vi "K线诊断.vi"(9 "K线诊断":string[][](table)=[["ATI", "MW60K 190630 V3.3"], ["ATSP5", "ISO14230 FastInit"], ["ATSH8131F1", "OK"], ["8100", "7F 81 13"]], 10 "波特率":u32=38400, 11 "VISA resource name":refnum<visa-resource-name> caption="COM") -> (2 "字符串":string, 3 "逻辑与":bool)   [LabVIEW 2020]
uses:
  <vilib>/Instr/_visa.llb/VISA Configure Serial Port (Instr).vi
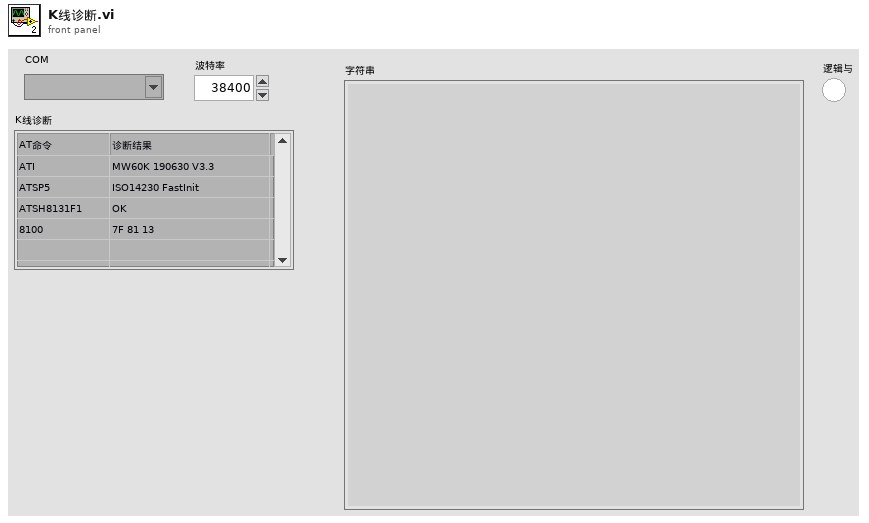
[diagram p1: front panel]
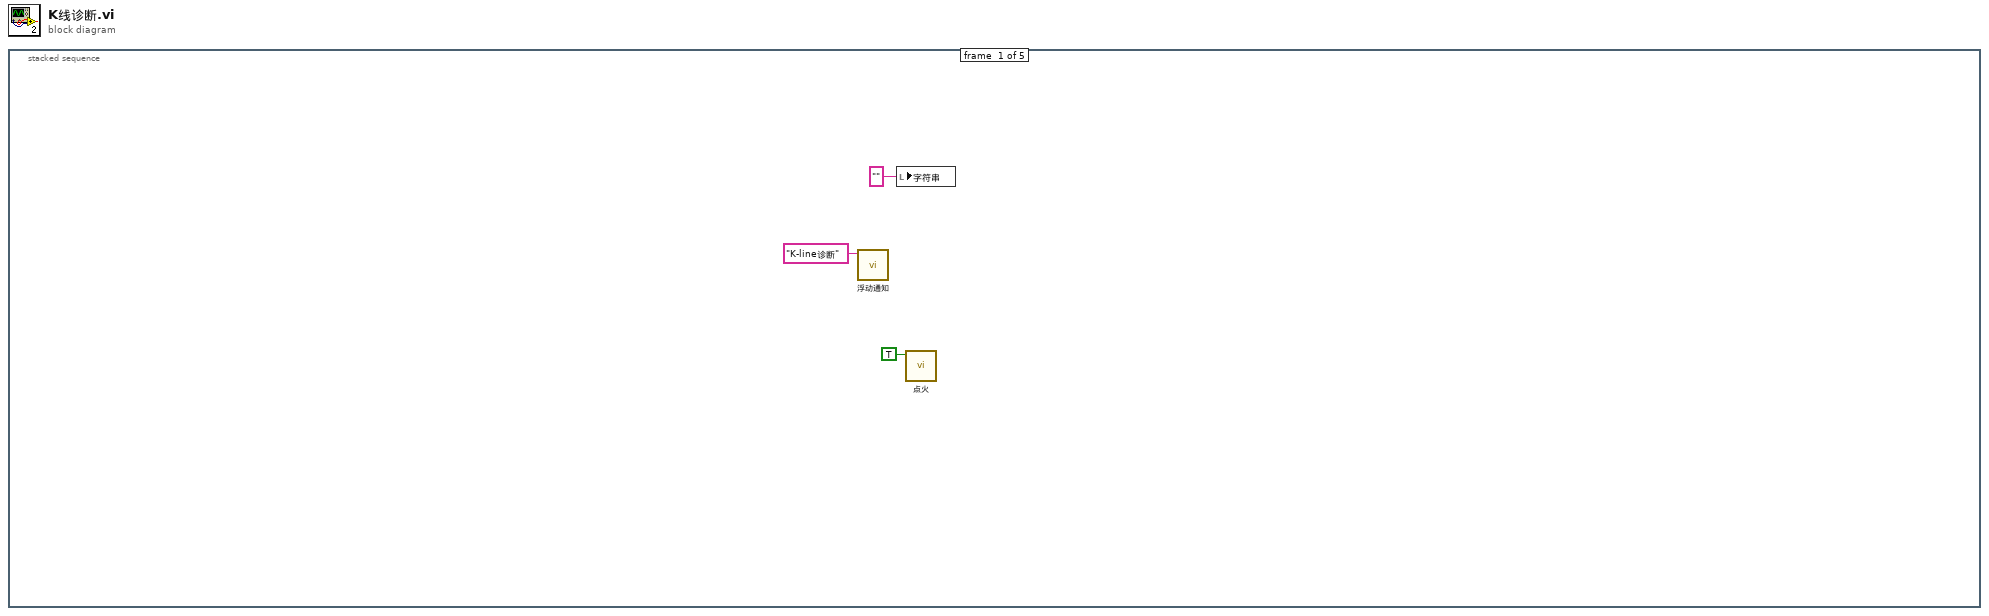
[diagram p0: block diagram]
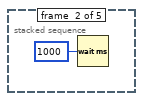
[diagram p2: hidden frame]
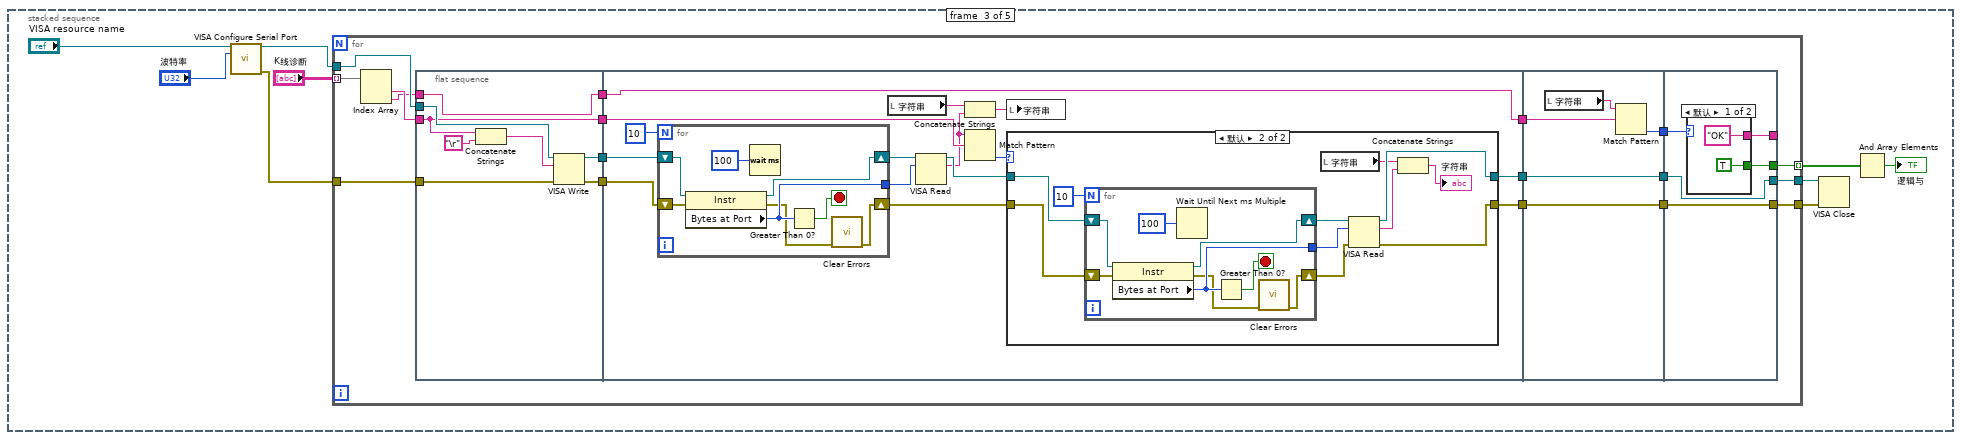
[diagram p3: hidden frame]
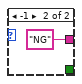
[diagram p5: hidden frame]
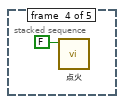
[diagram p6: hidden frame]
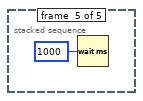
[diagram p7: hidden frame]
diagram:
  n1 = stacked-sequence {
    frame #0 {
      n2 = call "浮动通知.vi"("通知内容"="K-line诊断") -> ()  [unwired: 11 in]
      n3 = local write "字符串"("" ("字符串")) -> ()
      n4 = call "点火.vi"("点火"=TRUE) -> ()  [unwired: 10 in, 1 out]
    }
    frame #1 {
      n5 = Wait (ms)(milliseconds to wait=u32 1000 ("等待时间（毫秒）")) -> ()  [unwired: 1 out]
    }
    frame #2 {
      n6 = call-poly "VISA Configure Serial Port"("VISA resource name"="VISA resource name", "baud rate (9600)"="波特率") -> ("VISA resource name out"=w10:refnum<visa-resource-name>, "error out"=w9:errorcluster)  [unwired: 12 in]
      n7 = for {
        tunnel: "K线诊断" -> [w14] mode=indexing
        tunnel: w10 -> [w31]
        tunnel: w9 -> [w29]
        tunnel: [w23] -> w8
        tunnel: [w20] -> w7
        tunnel: [w15] -> w6 mode=indexing
        n8 = Index Array(array=w14) -> (element #1=w30:string, element #2=w28:string)  [unwired: 2 in]
        n9 = flat-sequence {
          tunnel: w31 -> [w39]
          tunnel: w30 -> [w32]
          tunnel: w29 -> [w37]
          tunnel: [w38] -> w19
          tunnel: [w36] -> w18
          tunnel: w28 -> [w33]
          tunnel: [w33] -> w17
          tunnel: [w32] -> w16
          tunnel: w19 -> [w51]
          tunnel: w18 -> [w40]
          tunnel: [w54] -> w27
          tunnel: w17 -> [w54]
          tunnel: [w53] -> w25
          tunnel: [w52] -> w22
          tunnel: w16 -> [w47]
          tunnel: w27 -> [w88]
          tunnel: [w87] -> w26
          tunnel: w25 -> [w86]
          tunnel: [w86] -> w24
          tunnel: w22 -> [w85]
          tunnel: [w85] -> w21
          tunnel: w26 -> [w93]
          tunnel: w24 -> [w91]
          tunnel: w21 -> [w90]
          tunnel: [w92] -> _
          tunnel: [w91] -> w23
          tunnel: [w90] -> w20
          tunnel: [w89] -> w15
          frame #0 {
            n10 = Concatenate Strings(w32, "\r") -> (w35:string)
            n11 = VISA Write(VISA resource name=w39, write buffer=w35, error in (no error)=w37) -> (VISA resource name out=w38:refnum<visa-resource-name>, error out=w36:errorcluster)  [unwired: 1 out]
          }
          frame #1 {
            n12 = for {
              N: 10 -> [_]
              tunnel: [w60] -> w50
              shift-right: [w61] -> w49
              shift-left: w51 -> [w62]
              shift-right: [w56] -> w41
              shift-left: w40 -> [w57]
              stop <- w59 stop-if-true
              n13 = property class="Instr"(reference=w62, error in=w57) -> (reference out=w61:refnum<visa-resource-name>, error out=w58:errorcluster, "Bytes at Port"=w60:u32)
              n14 = Wait (ms)(milliseconds to wait=u32 100 ("等待时间（毫秒）")) -> ()  [unwired: 1 out]
              n15 = Greater Than 0?(x=w60) -> (x > 0?=w59:bool)
              n16 = call <vilib>:"Clear Errors.vi"("error in (no error)"=w58) -> ("error out"=w56:errorcluster)  [unwired: 5 in, 1 out]
            }
            n17 = local read "字符串"() -> (w45:string)
            n18 = VISA Read(VISA resource name=w49, byte count=w50) -> (VISA resource name out=w48:refnum<visa-resource-name>, read buffer=w44:string)  [unwired: 1 in, 2 out]
            n19 = Concatenate Strings(w45, w44) -> (w43:string)
            n20 = Match Pattern(string=w44, regular expression=w47) -> (offset past match=w46:i32)  [unwired: 1 in, 3 out]
            n21 = local write "字符串"(w43) -> ()
            n22 = case shown="默认" w46 {
              tunnel: [w64 w73] -> w53
              tunnel: [w63 w72] -> w52
              tunnel: w41 -> [w63 w71]
              tunnel: w48 -> [w64 w68]
              frame -1 {
              }
              frame Default {
                n23 = for {
                  N: 10 -> [_]
                  tunnel: [w81] -> w74
                  shift-right: [w82] -> w75
                  shift-left: w68 -> [w83]
                  shift-right: [w78] -> w70
                  shift-left: w71 -> [w80]
                  stop <- w76 stop-if-true
                  n24 = property class="Instr"(reference=w83, error in=w80) -> (reference out=w82:refnum<visa-resource-name>, error out=w79:errorcluster, "Bytes at Port"=w81:u32)
                  n25 = Wait Until Next ms Multiple(millisecond multiple=u32 100 ("毫秒倍数")) -> ()  [unwired: 1 out]
                  n26 = Greater Than 0?(x=w81) -> (x > 0?=w76:bool)
                  n27 = call <vilib>:"Clear Errors.vi"("error in (no error)"=w79) -> ("error out"=w78:errorcluster)  [unwired: 5 in, 1 out]
                }
                n28 = local read "字符串"() -> (w66:string)
                n29 = VISA Read(VISA resource name=w75, byte count=w74, error in (no error)=w70) -> (VISA resource name out=w73:refnum<visa-resource-name>, read buffer=w65:string, error out=w72:errorcluster)  [unwired: 1 out]
                n30 = Concatenate Strings(w66, w65) -> (→"字符串":string)
              }
            }
          }
          frame #2 {
            n31 = local read "字符串"() -> (w84:string)
            n32 = Match Pattern(string=w84, regular expression=w88) -> (offset past match=w87:i32)  [unwired: 1 in, 3 out]
          }
          frame #3 {
            n33 = case shown="默认" w93 {
              tunnel: ["OK" "NG"] -> w92
              tunnel: [TRUE _] -> w89
              frame Default {
              }
              frame -1 {
              }
            }
          }
        }
      }
      n34 = VISA Close(VISA resource name=w8, error in (no error)=w7) -> ()  [unwired: 1 out]
      n35 = And Array Elements(Boolean array=w6) -> (logical AND=→"逻辑与":bool)
    }
    frame #3 {
      n36 = call "点火.vi"("点火"=FALSE) -> ()  [unwired: 10 in, 1 out]
    }
    frame #4 {
      n37 = Wait (ms)(milliseconds to wait=u32 1000 ("等待时间（毫秒）")) -> ()  [unwired: 1 out]
    }
  }
